vi "Loop_Timing_Slow_Loop.vi"(8 "error in":errorcluster, 11 "Controller Select":T1(ring)=enum."100hz/100hz" caption="Enum") -> (0 "error out":errorcluster, 2 "Iteration Count":dbl, 3 "Change Control Counter":dbl, 4 "Hz":dbl format="%#_4g")   [LabVIEW 2014]
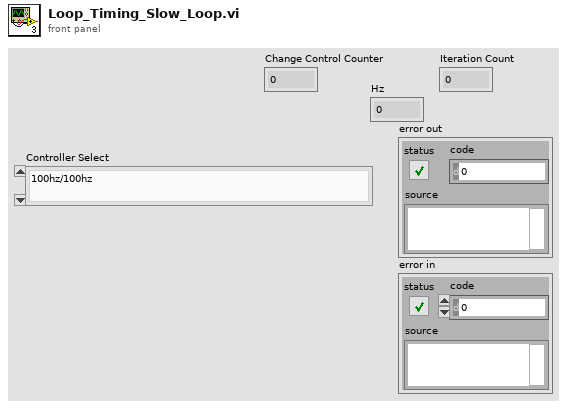
[diagram p1: front panel]
types:
  T1 = enum16{"100hz/50hz", "100hz/100hz", "200hz/200hz", "200hz/20hz", "User Defined"}
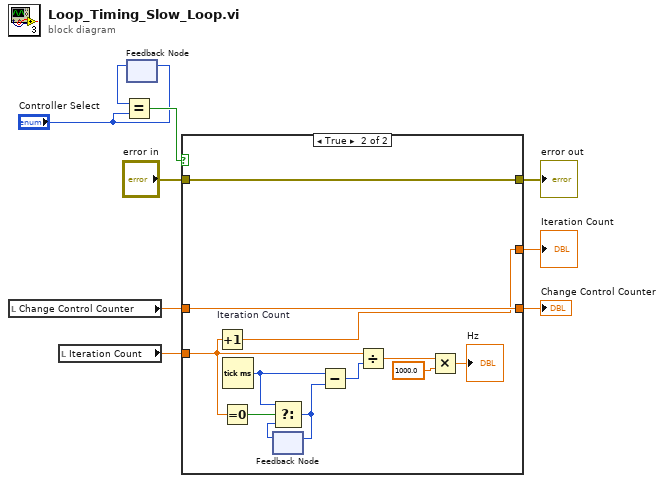
[diagram p0: block diagram]
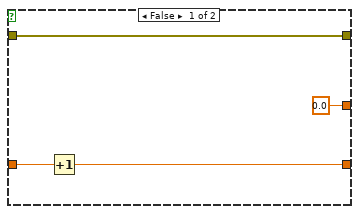
[diagram p2: hidden frame]
diagram:
  n1 = local read "Change Control Counter"() -> (w4:dbl)
  n2 = local read "Iteration Count"() -> (w2:dbl)
  n3 = feedback #1() -> (w6:T1)  [unwired: 1 in]
  n4 = Equal?(x=w6, y="Controller Select") -> (x = y?=w7:bool)
  n5 = feedback-in #1("Controller Select") -> ()
  n6 = case shown="True" w7 {
    tunnel: "error in" -> [w13 w17]
    tunnel: [w13 w17] -> w8
    tunnel: [w12 w16] -> w5
    tunnel: w4 -> [w11 w16]
    tunnel: [0.0 ("Iteration Count") w15] -> w3
    tunnel: w2 -> [_ w14]
    frame False {
      n7 = Increment(x=w11) -> (x+1=w12:dbl)
    }
    frame True {
      n8 = Increment "Iteration Count"(x=w14) -> (x+1=w15:dbl)
      n9 = Equal To 0?(x=w14) -> (x = 0?=w22:bool)
      n10 = Tick Count (ms)() -> (millisecond timer value=w21:u32)
      n11 = feedback #2() -> (w20:u32)  [unwired: 1 in]
      n12 = Select(t=w21, s=w22, f=w20) -> (s? t:f=w19:u32)
      n13 = feedback-in #2(w19) -> ()
      n14 = Subtract(x=w21, y=w19) -> (x-y=w18:u32)
      n15 = Divide(x=w14, y=w18) -> (x/y=w24:dbl)
      n16 = Multiply(x=w24, y=1000.0) -> (x*y=→"Hz":dbl)
    }
  }
  "error out" <- w8
  "Change Control Counter" <- w5
  "Iteration Count" <- w3
